vi "Fail.vi"() -> ()   [LabVIEW 2017, in "Caraya Test Framework.Tests.lvlib"]
uses:
  Caraya Test Framework.Tests.lvlib
  <vilib>/Utility/error.llb/Error Cluster From Error Code.vi
  <vilib>/ErrorRing/Error Ring.xnode
  src/Transparent Assertions/Assertions/Assertions.lvlib
  <vilib>/addons/_JKI Toolkits/Caraya/classes/Test/Test.lvclass
panel:
  out "error out":errorcluster
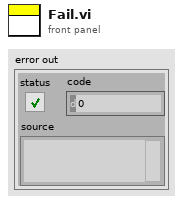
[diagram p1: front panel]
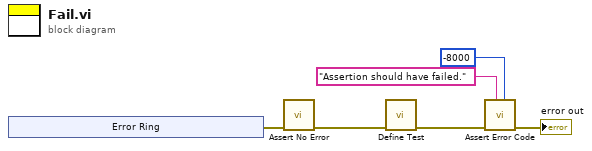
[diagram p0: block diagram]
diagram:
  n1 = xnode "Error Ring"() -> ("error out"=w6:errorcluster)
  n2 = call "Assert No Error.vi"("error in (no error)"=w6) -> ("error out"=w5:errorcluster)  [unwired: 10 in]
  n3 = call <vilib>:"Define Test.vi"("error in (no error)"=w5) -> ("error out"=w4:errorcluster)  [unwired: 9 in, 1 out]
  n4 = call "Assert Error Code.vi"("Expected"=-8000, "Message (\"\")"="Assertion should have failed." ("Message (\"\")"), "error in (no error)"=w4) -> ("error out"=→"error out":errorcluster)  [unwired: 8 in]
